vi "_error.vi"(8 "error in (no error)":errorcluster, 10 "Additional message":string, 11 "Status":T1) -> (0 "error out":errorcluster)   [LabVIEW 2013, in "tWorkerController.lvlib" / "tWorkerController.lvclass"]
uses:
  tWorkerController.lvclass
  _status.ctl
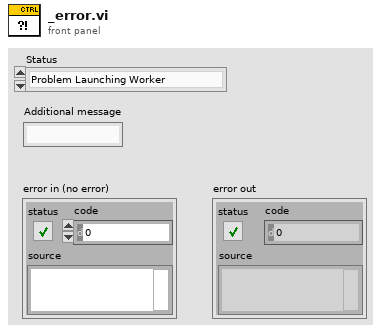
[diagram p1: front panel]
types:
  T1 = typedef "tWorkerController.lvlib/tWorkerController.lvclass/_status.ctl" = enum16{"Problem Launching Worker", "Worker Not Found", "Test Not In Library", "Connection Not Found"}
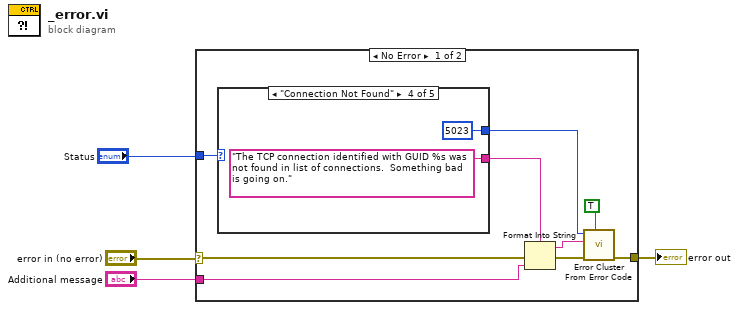
[diagram p0: block diagram]
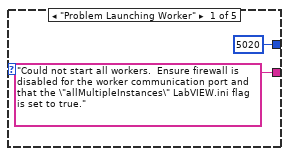
[diagram p2: hidden frame]
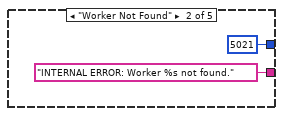
[diagram p3: hidden frame]
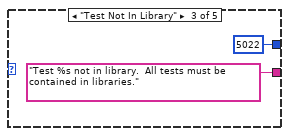
[diagram p4: hidden frame]
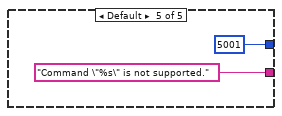
[diagram p5: hidden frame]
diagram:
  n1 = case shown="No Error" "error in (no error)" {
    selector: "error in (no error)" -> [w12 w24]
    tunnel: "Status" -> [w13 _]
    tunnel: "Additional message" -> [w10 _]
    tunnel: [w5 w24] -> w4
    frame No Error {
      n2 = case shown="\"Connection Not Found\"" w13 {
        tunnel: ["Could not start all workers.  Ensure firewall is disabled for the worker communication port and that the \"allMultipleInstances\" LabVIEW.ini flag is set to true." "INTERNAL ERROR: Worker %s not found." "Test %s not in library.  All tests must be contained in libraries." "The TCP connection identified with GUID %s was not found in list of connections.  Something bad is going on." "Command \"%s\" is not supported."] -> w11
        tunnel: [5020 5021 5022 5023 5001] -> w7
        frame "Problem Launching Worker" {
        }
        frame "Worker Not Found" {
        }
        frame "Test Not In Library" {
        }
        frame "Connection Not Found" {
        }
        frame Default {
        }
      }
      n3 = Format Into String(format string=w11, error in=w12, w10) -> (resulting string=w8:string, error out=w9:errorcluster)  [unwired: 1 in]
      n4 = call <vilib>:"Error Cluster From Error Code.vi"("show call chain? (False)"=TRUE, "error in (no error)"=w9, "error message (\"\")"=w8, "error code (0)"=w7) -> ("error out"=w5:errorcluster)  [unwired: 5 in]
    }
    frame Error {
    }
  }
  "error out" <- w4
